vi "AdventCode_Init.vi"(8 "Error In":errorcluster, 9 "Day":i32=2020, 10 "Year":i32=2020, 11 "reference in":refnum<class "AdventCode.lvclass"> caption="This control should only be used when\na sub class is inheriting this class") -> (0 "Error Out":errorcluster, 2 "PuzzleAvailable":bool, 3 "reference out":refnum<class "AdventCode.lvclass"> caption="This indicator should only be used when\na sub class is inheriting this class")   [LabVIEW 2020, in "AdventCode.lvclass"]
uses:
  AdventCode.lvclass
  AdventCode.lvclass/AdventCode.ctl
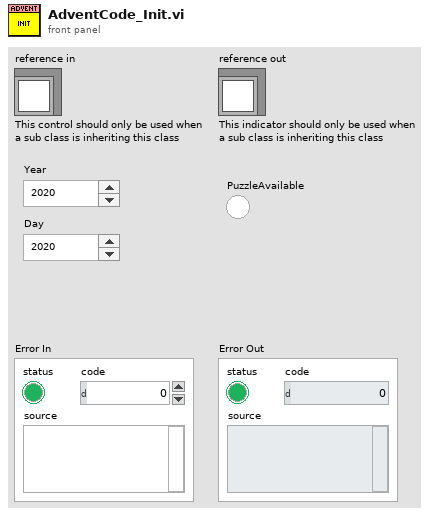
[diagram p1: front panel]
types:
  T1 = typedef "Puzzle.lvclass/ObjectAttributes.ctl" = cluster{"Year":i32, "Day":i32, "PuzzleData":string}
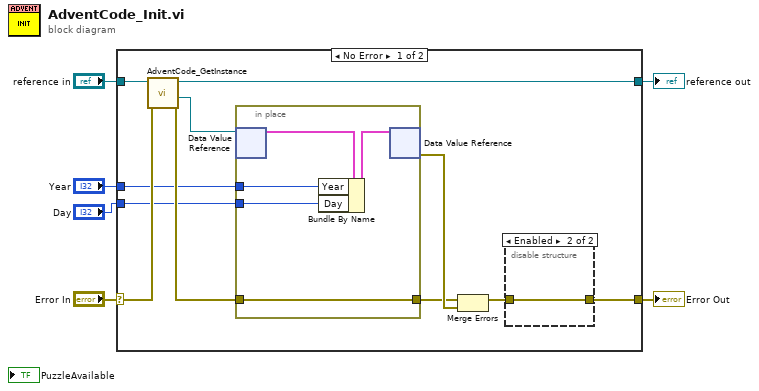
[diagram p0: block diagram]
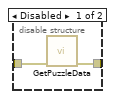
[diagram p2: hidden frame]
diagram:
  n1 = case shown="No Error" "Error In" {
    selector: "Error In" -> [w16 w27]
    tunnel: [w7 w27] -> w5
    tunnel: "reference in" -> [w15 w26]
    tunnel: [w13 w26] -> w3
    tunnel: "Year" -> [w10 _]
    tunnel: "Day" -> [w9 _]
    frame No Error {
      n2 = call "AdventCode_GetInstance.vi"("error in"=w16, "reference in"=w15) -> ("error out"=w12:errorcluster, "DVRRefOut"=w14:refnum<data-value>, "reference out"=w13:refnum<class "AdventCode.lvclass">)  [unwired: 5 in, 2 out]
      n3 = in-place {
        in-place-border: w12 -> [w23]
        in-place-border: [w23] -> w11
        in-place-border: w10 -> [w22]
        in-place-border: w9 -> [w21]
        n4 = in-place-dvr #1(w14) -> (w24:T1)  [unwired: 1 out]
        n5 = Bundle By Name(cluster=w24, "Year"=w22, "Day"=w21) -> (w25:T1)
        n6 = in-place-dvr #1(w25) -> (w17:errorcluster)  [unwired: 1 out]
      }
      n7 = Merge Errors(w11, w17) -> (w8:errorcluster)
      n8 = disable-structure shown="Enabled" {
        disable-tunnel: w8 -> [w19 w20]
        disable-tunnel: [w18 w20] -> w7
        frame Disabled {
          n9 = call "GetPuzzleData.vi"("Error In"=w19) -> ("Error Out"=w18:errorcluster)  [unwired: 10 in]
        }
        frame Enabled {
        }
      }
    }
    frame Error {
    }
  }
  "Error Out" <- w5
  "reference out" <- w3
